vi "QuVI_Wire (added).vi"(2 "Stack in":refnum<class "QuSim.lvclass">) -> (8 "QuWire out":refnum<class "QuWire.lvclass">, 13 "Stack out":refnum<class "QuSim.lvclass">)   [LabVIEW 2020]
doc: "Initializes a qubit in the state |0> and provides a reference wire for circuit construction.\n\nTo build a multi-qubit register, stack multiple instances of this VI vertically on the block diagram. The vertical connections aggregate the qubit count for the global state vector.\n\nTerminals:\n\n[Top] Stack in: Connect from the 'Stack out' of the previous qubit above. \n\n[Bottom] Stack out: Connect to the 'Stack in' of the next qubit below.\n\n[Right] Quantum Wire Ref: The \"QuWire.\" Connect this to the left border of a Flat Sequence Structure."
uses:
  QuSim.lvclass
  QuWire/QuWire.lvclass
  C:/Users/HP/OneDrive/LabVIEW/Quantum Circuit Simulator/VIPM/QuVI 2020/QuSim/QuSim.lvclass
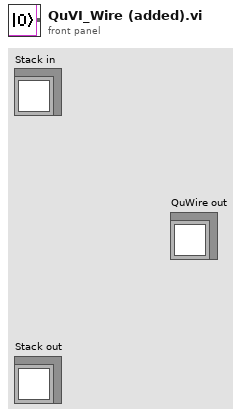
[diagram p1: front panel]
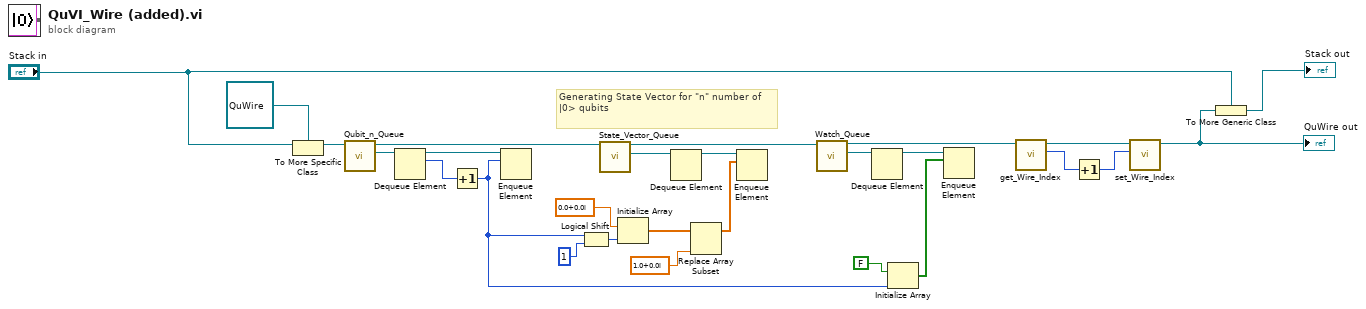
[diagram p0: block diagram]
diagram:
  # "Generating State Vector for \"n\" number of |0> qubits"
  n1 = To More Specific Class(target class=refnum<class "QuWire.lvclass"> refnum ("Wire.lvclass"), reference="Stack in") -> (specific class reference=w23:refnum<class "QuWire.lvclass">)  [unwired: 1 in, 1 out]
  n2 = call "Qubit_n_Queue.vi"("QuWire in"=w23) -> ("Qubit n"=w24:refnum<queue>, "QuWire out"=w6:refnum<class "QuWire.lvclass">)  [unwired: 8 in, 1 out]
  n3 = Dequeue Element(queue=w24) -> (queue out=w25:refnum<queue>, element=w26:i32)  [unwired: 2 in, 2 out]
  n4 = Increment(x=w26) -> (x+1=w7:i32)
  n5 = Enqueue Element(queue=w25, element=w7) -> ()  [unwired: 2 in, 3 out]
  n6 = Logical Shift(y=w7, x=u32 1) -> (x << y=w11:u32)
  n7 = call "State_Vector_Queue.vi"("QuWire in"=w6) -> ("State Vector Queue"=w14:refnum<queue>, "QuWire out"=w4:refnum<class "QuWire.lvclass">)  [unwired: 8 in, 1 out]
  n8 = Initialize Array(cdb 0.0+0.0i ("element"), w11) -> (w10:cdb[])
  n9 = Dequeue Element(queue=w14) -> (queue out=w15:refnum<queue>)  [unwired: 2 in, 3 out]
  n10 = Replace Array Subset(array=w10, new element=cdb 1.0+0.0i ("element")) -> (w8:cdb[])  [unwired: 1 in]
  n11 = Enqueue Element(queue=w15, element=w8) -> ()  [unwired: 2 in, 3 out]
  n12 = call "Watch_Queue.vi"("QuWire in"=w4) -> ("Watch List"=w17:refnum<queue>, "QuWire out"=w5:refnum<class "QuWire.lvclass">)  [unwired: 8 in, 1 out]
  n13 = Dequeue Element(queue=w17) -> (queue out=w18:refnum<queue>)  [unwired: 2 in, 3 out]
  n14 = Initialize Array(FALSE, w7) -> (w19:bool[])
  n15 = Enqueue Element(queue=w18, element=w19) -> ()  [unwired: 2 in, 3 out]
  n16 = call "get_Wire_Index.vi"("QuWire in"=w5) -> ("Wire Index"=w21:i32, "QuWire out"=w20:refnum<class "QuWire.lvclass">)  [unwired: 8 in, 1 out]
  n17 = Increment(x=w21) -> (x+1=w22:i32)
  n18 = call "set_Wire_Index.vi"("Wire Index"=w22, "QuWire in"=w20) -> ("QuWire out"=w3:refnum<class "QuWire.lvclass">)  [unwired: 8 in, 1 out]
  "QuWire out" <- w3
  n19 = To More Generic Class(target class="Stack in", reference=w3) -> (generic class reference=→"Stack out":refnum<class "QuSim.lvclass">)
